vi "DeInit Done.vi"(8 "error in (no error)":errorcluster, 9 "Initialized":bool, 10 "InstrumentData":T1={"Instr Error"={"status"=FALSE, "code"=0, "source"=""}, "Address"={"address type"=enum."VISA", "Address"="", "instrument type"=enum."Spectrometer"}, "CurrentState"={"Initialized"=FALSE, "Connected"=FALSE, "Running"=FALSE, "Error"=FALSE}}, 11 "SpectrumAnalyzerUI.lvclass":refnum<class "SpectrumAnalyzerUI.lvclass">) -> (0 "error out":errorcluster, 3 "SpectrumAnalyzerUI.lvclass":refnum<class "SpectrumAnalyzerUI.lvclass">)   [LabVIEW 2023, in "SpectrumAnalyzerUI.lvlib" / "SpectrumAnalyzerUI.lvclass"]
uses:
  typedefs/InstrumentData.ctl
  typedefs/instrumentType.ctl
  SpectrumAnalyzerUI.lvclass
  SpectrumAnalyzerUI.lvclass/SpectrumAnalyzerUI.ctl
  typedefs/typedefs.lvlib
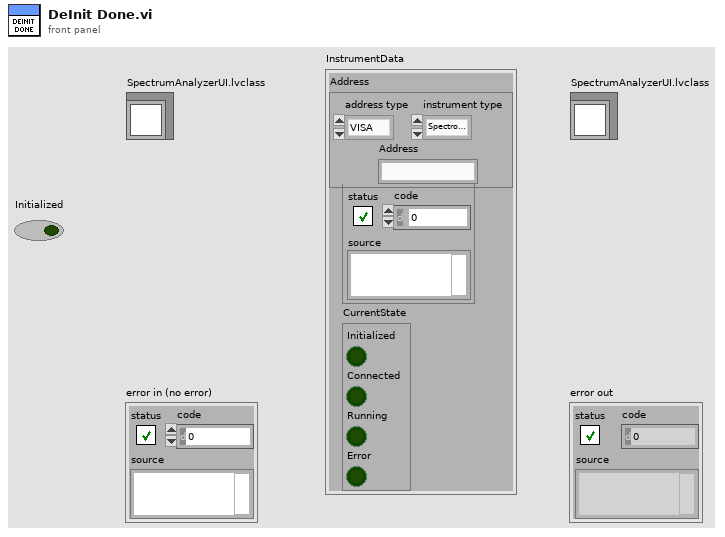
[diagram p1: front panel]
types:
  T1 = typedef "typedefs.lvlib/InstrumentData.ctl" = cluster{"Instr Error":errorcluster, "Address":cluster{"address type":enum16{"VISA", "Index"}, "Address":string, "instrument type":T2}, "CurrentState":cluster{"Initialized":bool, "Connected":bool, "Running":bool, "Error":bool}}
  T2 = typedef "typedefs.lvlib/instrumentType.ctl" = enum16{"Spectrum Analyzer", "Spectrometer", "Camera", "Stepper", "Piezo", "SLM"}
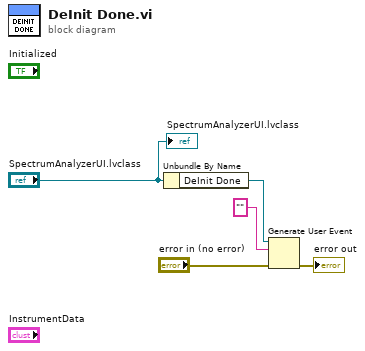
[diagram p0: block diagram]
diagram:
  n1 = Unbundle By Name("SpectrumAnalyzerUI.lvclass") -> ("DeInit Done"=w4:refnum<user-event>)
  n2 = Generate User Event(user event=w4, event data cluster="" ("event data"), error in="error in (no error)") -> (error out=→"error out":errorcluster)  [unwired: 1 in, 1 out]
  "SpectrumAnalyzerUI.lvclass" <- "SpectrumAnalyzerUI.lvclass"
